vi "18.DMA-FIFO-2通道 (Host).vi"() -> ()   [LabVIEW 2019]
uses:
  <vilib>/rvi/interface/nirviOpenFPGA/nirviOpenFPGA.xnode
  <vilib>/rvi/interface/nirviMethod/nirviMethod.xnode
  <vilib>/rvi/errors/niLvFpgaMergeErrorWithErrorCode.vi
  <vilib>/FPGAPlugInAG/ELVIS III/niLvFpga_ReadFifo_ELVIS III.vi
  <vilib>/rvi/interface/nirviReadWriteControl/nirviReadWriteControl.xnode
  <vilib>/Utility/error.llb/Error Cluster From Error Code.vi
  <vilib>/rvi/errors/niLvFpgaAdjustHostInterfaceError.vi
  NiFpgaLv.dll
  <vilib>/rvi/interface/nirviCloseFPGA/nirviCloseFPGA.xnode
  <vilib>/FPGAPlugInAG/ELVIS III/niLvFpga_Open_ELVIS III.vi
  <vilib>/FPGAPlugInAG/ELVIS III/niLvFpga_Reset_ELVIS III.vi
  <vilib>/FPGAPlugInAG/ELVIS III/niLvFpga_ConfigureFifo_ELVIS III.vi
  <vilib>/FPGAPlugInAG/ELVIS III/niLvFpga_Run_ELVIS III.vi
  <vilib>/FPGAPlugInAG/ELVIS III/niLvFpga_Close_ELVIS III.vi
panel:
  out "错误输出":errorcluster
  in  "stop":bool
  out "Overflow Count":u32
  out "Accelerometer Data":dbl[][](graph)
  in  "Samples per Channel":u32=1000
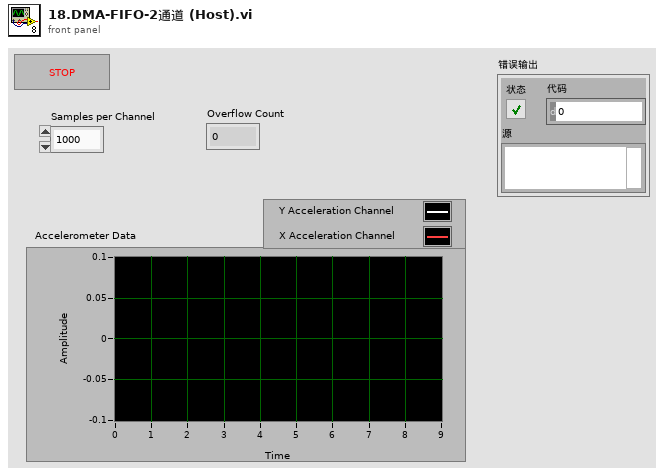
[diagram p1: front panel]
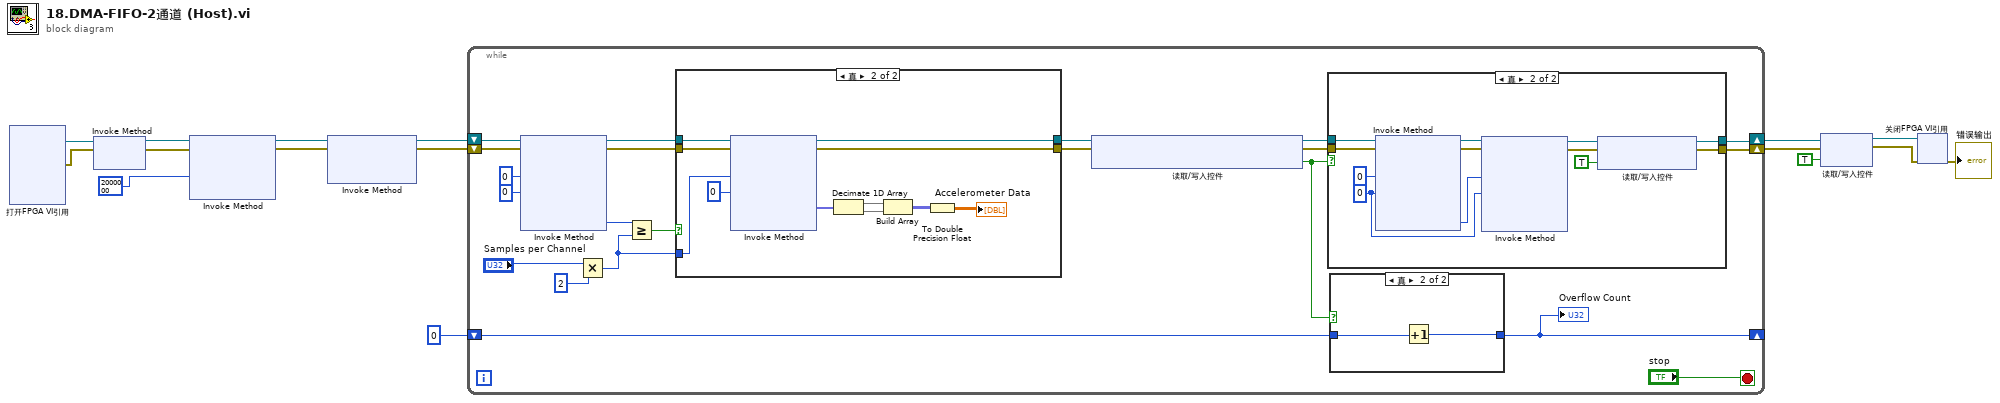
[diagram p0: block diagram]
diagram:
  n1 = xnode "打开FPGA VI引用"() -> ("FPGA VI引用输出"=w15:refnum<k20>, "错误输出"=w16:errorcluster)  [unwired: 2 in]
  n2 = xnode "Invoke Method"("FPGA VI引用输入"=w15, "错误输入"=w16) -> ("FPGA VI引用输出"=w13:refnum<k20>, "错误输出"=w14:errorcluster)
  n3 = xnode "Invoke Method"("FPGA VI引用输入"=w13, "错误输入"=w14, "请求的深度"=u32 2000000 ("Depth")) -> ("FPGA VI引用输出"=w10:refnum<k20>, "错误输出"=w11:errorcluster)  [unwired: 1 out]
  n4 = xnode "Invoke Method"("FPGA VI引用输入"=w10, "错误输入"=w11) -> ("FPGA VI引用输出"=w9:refnum<k20>, "错误输出"=w8:errorcluster)  [unwired: 1 in]
  n5 = while {
    shift-right: [w22] -> w6
    shift-left: w8 -> [w37]
    shift-right: [w21] -> w5
    shift-left: w9 -> [w36]
    shift-right: [w18] -> _
    shift-left: u32 0 -> [w19]
    stop <- "stop" stop-if-true
    n6 = xnode "Invoke Method"("FPGA VI引用输入"=w36, "错误输入"=w37, "元素数量"=u32 0, "超时(ms)"=0) -> ("FPGA VI引用输出"=w28:refnum<k20>, "错误输出"=w29:errorcluster, "剩余元素"=w33:u32)  [unwired: 1 out]
    n7 = Multiply(x="Samples per Channel", y=u32 2) -> (x*y=w27:u32)
    n8 = Greater Or Equal?(x=w33, y=w27) -> (x >= y?=w30:bool)
    n9 = case shown="真" w30 {
      tunnel: w29 -> [w56 w66]
      tunnel: w28 -> [w55 w67]
      tunnel: w27 -> [_ w64]
      tunnel: [w56 w58] -> w26
      tunnel: [w55 w57] -> w25
      frame False {
      }
      frame True {
        n10 = xnode "Invoke Method"("FPGA VI引用输入"=w67, "错误输入"=w66, "元素数量"=w64, "超时(ms)"=0) -> ("FPGA VI引用输出"=w57:refnum<k20>, "错误输出"=w58:errorcluster, "数据"=w63:fxp<+/-,24,5>[])  [unwired: 1 out]
        n11 = Decimate 1D Array(w63) -> (w62:fxp<+/-,24,5>[], w61:fxp<+/-,24,5>[])
        n12 = Build Array(w62, w61) -> (w60:fxp<+/-,24,5>[][])
        n13 = To Double Precision Float(number=w60) -> (double precision float=→"Accelerometer Data":dbl[][])
      }
    }
    n14 = xnode "读取/写入控件"("FPGA VI引用输入"=w25, "错误输入"=w26) -> ("FPGA VI引用输出"=w23:refnum<k20>, "错误输出"=w24:errorcluster, "Overflow?"=w20:bool)
    n15 = case shown="真" w20 {
      tunnel: w24 -> [w42 w54]
      tunnel: w23 -> [w41 w53]
      tunnel: [w42 w44] -> w22
      tunnel: [w41 w43] -> w21
      frame False {
      }
      frame True {
        w48 = 0 ("超时(ms)")
        n16 = xnode "Invoke Method"("FPGA VI引用输入"=w53, "错误输入"=w54, "元素数量"=u32 0, "超时(ms)"=w48) -> ("FPGA VI引用输出"=w50:refnum<k20>, "错误输出"=w51:errorcluster, "剩余元素"=w49:u32)  [unwired: 1 out]
        n17 = xnode "Invoke Method"("FPGA VI引用输入"=w50, "错误输入"=w51, "元素数量"=w49, "超时(ms)"=w48) -> ("FPGA VI引用输出"=w46:refnum<k20>, "错误输出"=w47:errorcluster)  [unwired: 2 out]
        n18 = xnode "读取/写入控件"("FPGA VI引用输入"=w46, "错误输入"=w47, "DMA Cleared?"=TRUE) -> ("FPGA VI引用输出"=w43:refnum<k20>, "错误输出"=w44:errorcluster)
      }
    }
    n19 = case shown="真" w20 {
      tunnel: w19 -> [w38 w40]
      tunnel: [w38 w39] -> w18
      frame False {
      }
      frame True {
        n20 = Increment(x=w40) -> (x+1=w39:u32)
      }
    }
    "Overflow Count" <- w18
  }
  n21 = xnode "读取/写入控件"("FPGA VI引用输入"=w5, "错误输入"=w6, "stop"=TRUE) -> ("FPGA VI引用输出"=w3:refnum<k20>, "错误输出"=w2:errorcluster)
  n22 = xnode "关闭FPGA VI引用"("FPGA VI引用输入"=w3, "错误输入"=w2) -> ("错误输出"=→"错误输出":errorcluster)
